vi "sv_Check for Weighting Change (time signal).vi"(6 "weighting":T1 items=["Linear", "A-weighting", "B-weighting", "C-weighting", "ITU-R 468-4", "Dolby", "CCITT", "C-message", "Wb", "Wc", "Wd", "We", "Wf", "Wh", "Wj", "Wk", "Wm", "AES17 20 kHz lowpass", "AES17 40 kHz lowpass", "AES17 20 kHz highpass", "AES17 40 kHz highpass"], 7 "reset (in)":bool, 8 "error in (no error)":errorcluster) -> (0 "error out":errorcluster, 1 "weighting has changed":bool, 4 "dup weighting":T1 items=["Linear", "A-weighting", "B-weighting", "C-weighting", "ITU-R 468-4", "Dolby", "CCITT", "C-message", "Wb", "Wc", "Wd", "We", "Wf", "Wh", "Wj", "Wk", "Wm", "AES17 20 kHz lowpass", "AES17 40 kHz lowpass", "AES17 20 kHz highpass", "AES17 40 kHz highpass"])   [LabVIEW 2017]
uses:
  <vilib>/addons/_NISVFA/_Shared subVIs/Controls/svc_Weighting Filter Text Ring.ctl
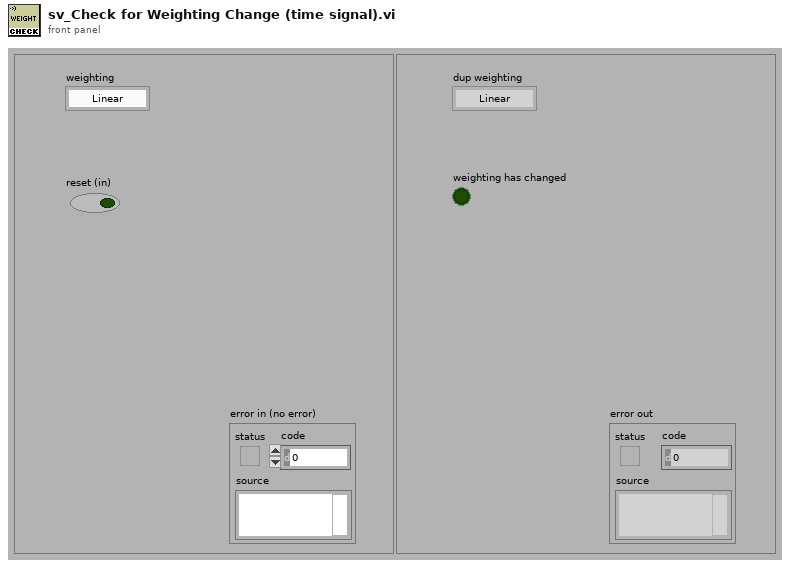
[diagram p1: front panel]
types:
  T1 = typedef "svc_Weighting Filter Text Ring.ctl" = u16
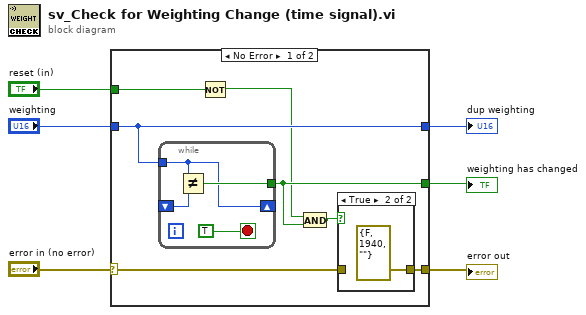
[diagram p0: block diagram]
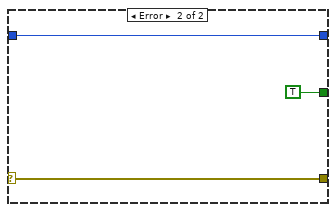
[diagram p3: hidden frame]
diagram:
  n1 = case shown="No Error" "error in (no error)" {
    selector: "error in (no error)" -> [w12 w21]
    tunnel: "weighting" -> [w13 w22]
    tunnel: [w11 w21] -> w4
    tunnel: [w13 w22] -> w3
    tunnel: [w8 TRUE] -> w2
    tunnel: "reset (in)" -> [w10 _]
    frame No Error {
      n2 = while {
        tunnel: [w16] -> w8
        tunnel: w13 -> [w14]
        shift-left: _ -> [w15]
        shift-right: [w14] -> _
        stop <- TRUE stop-if-true
        n3 = Not Equal?(x=w14, y=w15) -> (x != y?=w16:bool)
      }
      n4 = Not(x=w10) -> (.not. x?=w7:bool)
      n5 = And(x=w7, y=w8) -> (x .and. y?=w9:bool)
      n6 = case shown="True" w9 {
        tunnel: w12 -> [w18 _]
        tunnel: [w18 errorcluster {"status"=FALSE, "code"=1940, "source"=""} ("error IO")] -> w11
        frame False {
        }
        frame True {
        }
      }
    }
    frame Error {
    }
  }
  "error out" <- w4
  "dup weighting" <- w3
  "weighting has changed" <- w2
